vi "PPS Parse to type.vi"(5 "ClassName":string, 8 "error in (no error)":errorcluster, 9 "User's new value":string, 10 "Control name":string, 11 "Control in":refnum<vi>) -> (0 "error out":errorcluster, 3 "ack":string)   [LabVIEW 2016]
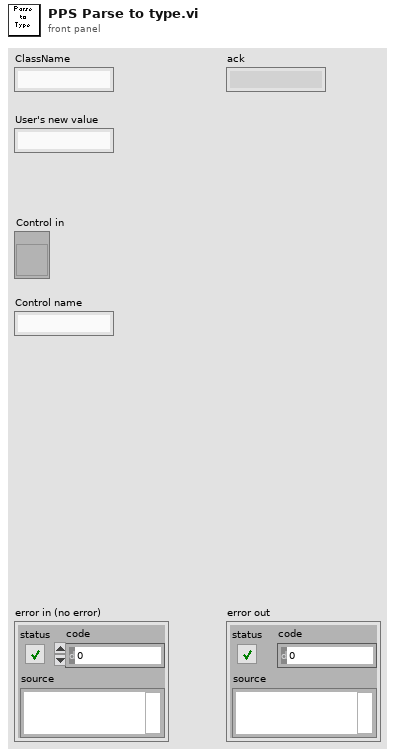
[diagram p1: front panel]
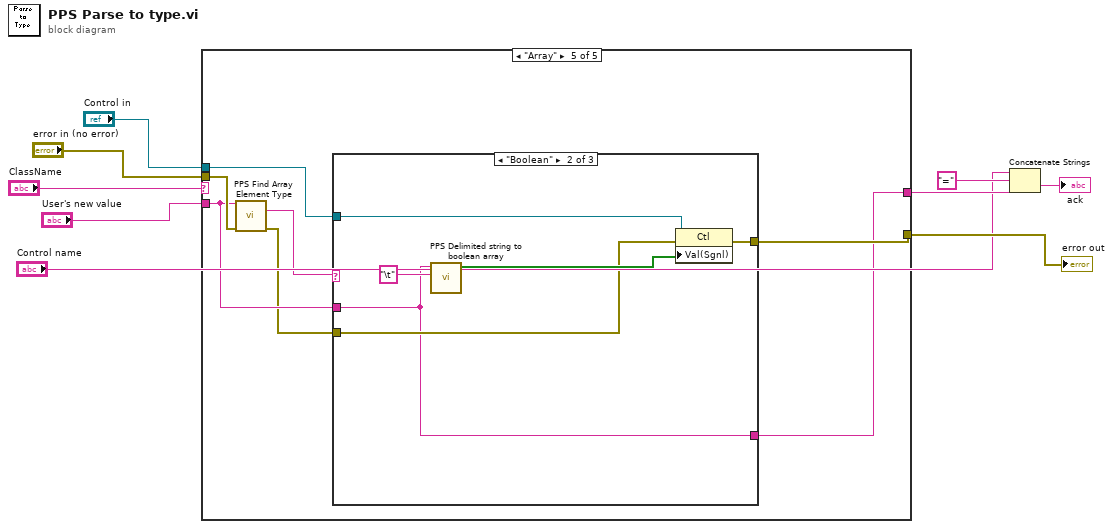
[diagram p0: block diagram]
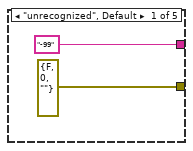
[diagram p2: hidden frame]
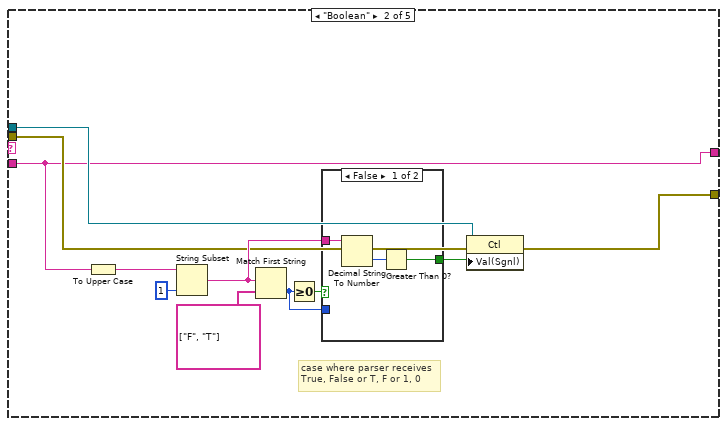
[diagram p3: hidden frame]
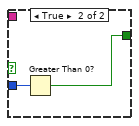
[diagram p4: hidden frame]
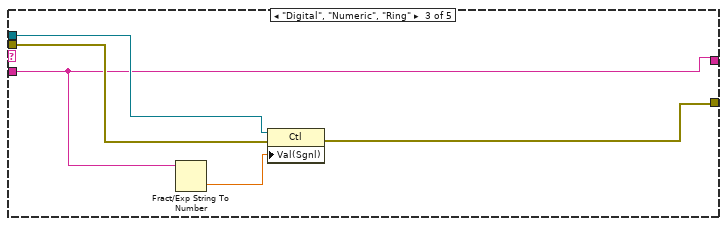
[diagram p5: hidden frame]
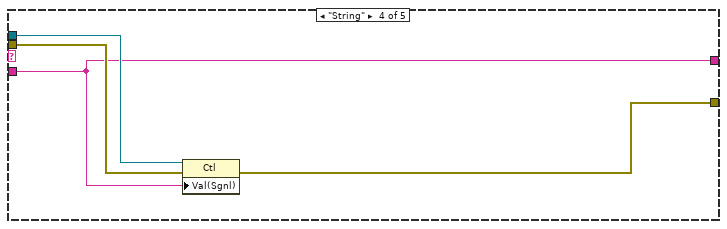
[diagram p6: hidden frame]
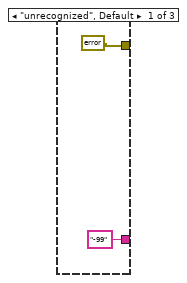
[diagram p7: hidden frame]
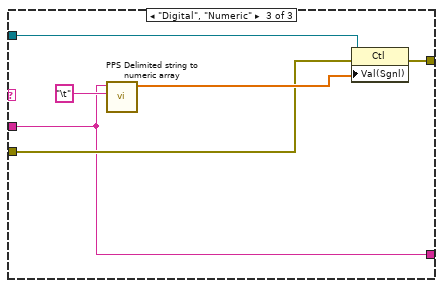
[diagram p8: hidden frame]
diagram:
  n1 = case shown="\"Array\"" "ClassName" {
    tunnel: [errorcluster {"status"=FALSE, "code"=0, "source"=""} ("error out") w13 w29 w34 w38] -> w6
    tunnel: "Control in" -> [_ w14 w31 w36 w42]
    tunnel: "error in (no error)" -> [_ w15 w30 w35 w43]
    tunnel: "User's new value" -> [_ w12 w28 w33 w40]
    tunnel: ["-99" w12 w28 w33 w37] -> w2
    frame "unrecognized", Default {
    }
    frame "Boolean" {
      # "case where parser receives\nTrue, False or T, F or 1, 0"
      n2 = To Upper Case(1:w12) -> (0:w18:string)
      n3 = String Subset(string=w18, length (rest)=1 ("length (rest)")) -> (substring=w16:string)  [unwired: 1 in]
      n4 = Match First String(2:string[] ["F", "T"] ("string array"), 3:w16) -> (0:w19:i32)  [unwired: 1 out]
      n5 = Greater Or Equal To 0?(x=w19) -> (x >= 0?=w20:bool)
      n6 = case shown="False" w20 {
        tunnel: w19 -> [_ w27]
        tunnel: w16 -> [w24 _]
        tunnel: [w23 w26] -> w22
        frame False {
          n7 = Decimal String To Number(string=w24) -> (number=w25:i32)  [unwired: 2 in, 1 out]
          n8 = Greater Than 0?(x=w25) -> (x > 0?=w23:bool)
        }
        frame True {
          n9 = Greater Than 0?(x=w27) -> (x > 0?=w26:bool)
        }
      }
      n10 = property class="Ctl"(reference=w14, error in=w15, "Val(Sgnl)"=w22) -> (error out=w13:errorcluster)  [unwired: 1 out]
    }
    frame "Digital", "Numeric", "Ring" {
      n11 = Fract/Exp String To Number(string=w28) -> (number=w32:dbl)  [unwired: 3 in, 1 out]
      n12 = property class="Ctl"(reference=w31, error in=w30, "Val(Sgnl)"=w32) -> (error out=w29:errorcluster)  [unwired: 1 out]
    }
    frame "String" {
      n13 = property class="Ctl"(reference=w36, error in=w35, "Val(Sgnl)"=w33) -> (error out=w34:errorcluster)  [unwired: 1 out]
    }
    frame "Array" {
      n14 = call "PPS Find Array Element Type.vi"("Variant"=w40, "error in (no error)"=w43) -> ("Element type Name"=w41:string, "error out"=w39:errorcluster)  [unwired: 9 in, 3 out]
      n15 = case shown="\"Boolean\"" w41 {
        tunnel: [errorcluster {"status"=FALSE, "code"=0, "source"=""} ("error in (no error)") w50 w56] -> w38
        tunnel: w39 -> [_ w47 w53]
        tunnel: w40 -> [_ w46 w52]
        tunnel: w42 -> [_ w51 w57]
        tunnel: ["-99" ("User's new value") w46 w52] -> w37
        frame "unrecognized", Default {
        }
        frame "Boolean" {
          n16 = call "PPS Delimited string to boolean array.vi"("delimiter"="\t", "1D string of Booleans separated by delimiter"=w46) -> ("Boolean array"=w48:bool[])  [unwired: 9 in]
          n17 = property class="Ctl"(reference=w51, error in=w47, "Val(Sgnl)"=w48) -> (error out=w50:errorcluster)  [unwired: 1 out]
        }
        frame "Digital", "Numeric" {
          n18 = call "PPS Delimited string to numeric array.vi"("delimiter"="\t", "1D string of numerics separated by delimiter"=w52) -> ("Float array"=w54:dbl[])  [unwired: 9 in]
          n19 = property class="Ctl"(reference=w57, error in=w53, "Val(Sgnl)"=w54) -> (error out=w56:errorcluster)  [unwired: 1 out]
        }
      }
    }
  }
  "error out" <- w6
  n20 = Concatenate Strings("Control name", "=" ("string"), w2) -> (→"ack":string)
